vi "ADI_IMU_ADIS16448_GetSetRefNum.vi"(8 "error in (no error)":errorcluster, 9 "menu":enum16{"set", "get"}(ring), 10 "refnum name":string, 11 "ADI IMU Interrupt DevRef Set":T1) -> (0 "error out":errorcluster, 3 "ADI IMU Interrupt DevRef Get":T1)   [LabVIEW 2016, in "ADIS16448_IMU.lvlib"]
doc: "Sets a reference into a registry, gets a reference from a registry, or deletes a reference from a registry. The reference is accessed by name, and can be given any unique name.\n\nThis software is licensed. Open the labview\\readme\\WPI Robotics Library Open Source License.txt file for more information."
uses:
  ADIS16448_IMU.lvlib
  ADI_IMU_ADIS16448_InterruptDevRef.ctl
  ADI_IMU_ADIS16448_IMUDevRef.ctl
  <vilib>/Rock Robotics/SystemInterfaces/spilib/spi_bus.ctl
  <vilib>/Rock Robotics/WPI/Interrupt/WPI_InterruptRef.ctl
  <vilib>/Rock Robotics/SystemInterfaces/Interrupt/FPGA_InterruptIndex.ctl
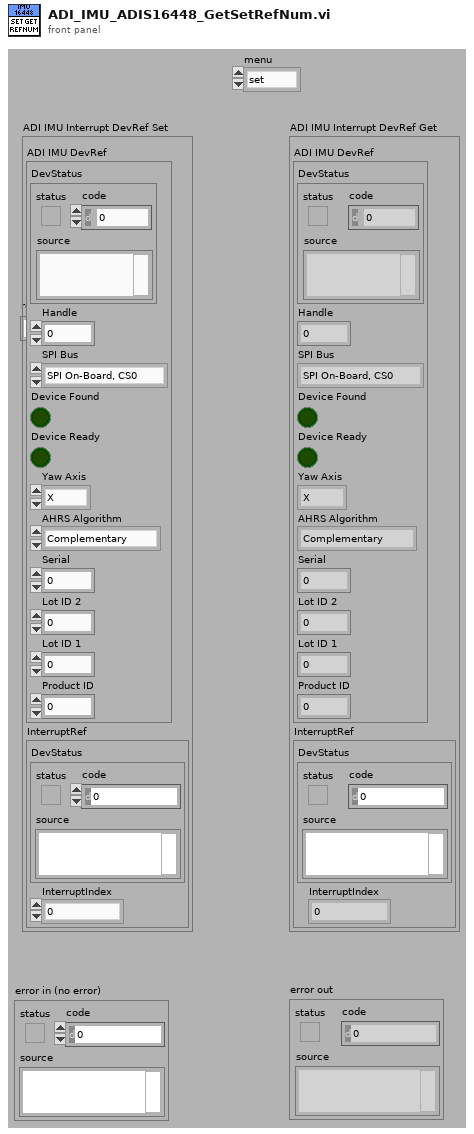
[diagram p1: front panel]
types:
  T1 = typedef "ADIS16448_IMU.lvlib/ADI_IMU_ADIS16448_InterruptDevRef.ctl" = cluster{"ADI IMU DevRef":T2, "InterruptRef":T4}
  T2 = typedef "ADIS16448_IMU.lvlib/ADI_IMU_ADIS16448_IMUDevRef.ctl" = cluster{"DevStatus":errorcluster, "Handle":i32, "SPI Bus":T3, "Device Found":bool, "Device Ready":bool, "Yaw Axis":enum16{"X", "Y", "Z"}, "AHRS Algorithm":enum16{"Complementary", "Madgwick"}, "Serial":u16, "Lot ID 2":u16, "Lot ID 1":u16, "Product ID":u16}
  T3 = typedef "spi_bus.ctl" = enum16{"SPI On-Board, CS0", "SPI On-Board, CS1", "SPI On-Board, CS2", "SPI On-Board, CS3", "SPI MXP", "Invalid"}
  T4 = typedef "WPI_InterruptRef.ctl" = cluster{"DevStatus":errorcluster, "InterruptIndex":T5}
  T5 = typedef "FPGA_InterruptIndex.ctl" = enum8{"0", "1", "2", "3", "4", "5", "6", "7", "Invalid"}
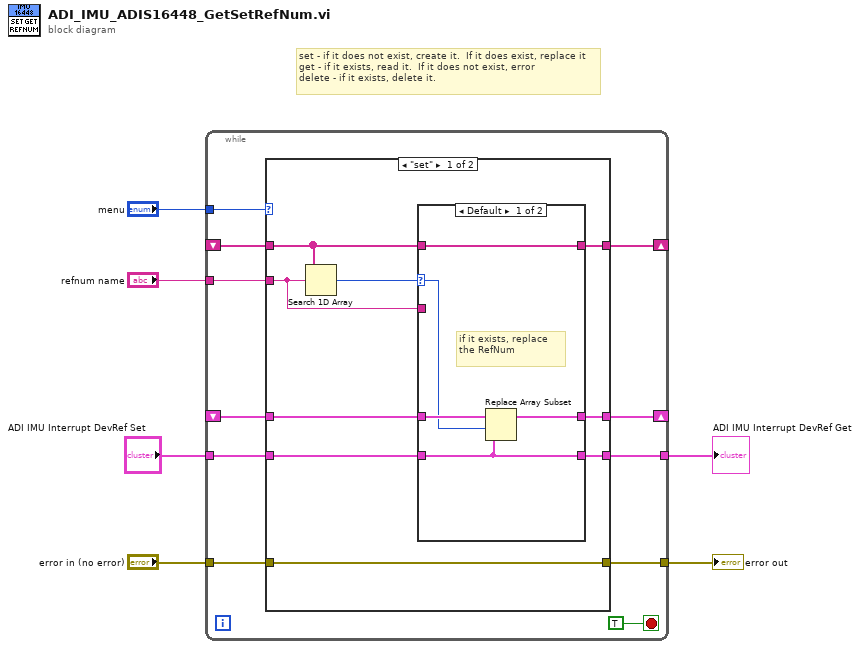
[diagram p0: block diagram]
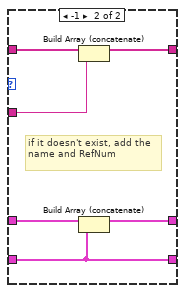
[diagram p2: hidden frame]
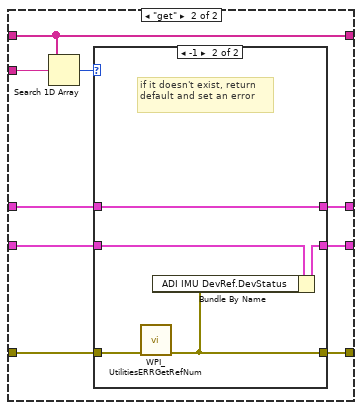
[diagram p3: hidden frame]
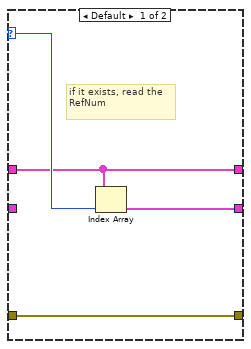
[diagram p4: hidden frame]
diagram:
  # "set - if it does not exist, create it.  If it does exist, replace it\nget - if it exists, read it.  If it does not exist, error\ndelete - if it exists, delete it."
  n1 = while {
    tunnel: "ADI IMU Interrupt DevRef Set" -> [w17]
    tunnel: "refnum name" -> [w10]
    tunnel: "error in (no error)" -> [w9]
    shift-right: [w16] -> _
    shift-left: _ -> [w15]
    tunnel: [w14] -> w1
    tunnel: "menu" -> [w13]
    shift-right: [w12] -> _
    shift-left: _ -> [w11]
    tunnel: [w8] -> w4
    stop <- TRUE stop-if-true
    n2 = case shown="\"set\"" w13 {
      tunnel: w17 -> [w21 w43]
      tunnel: [w20 w42] -> w16
      tunnel: w15 -> [w22 w44]
      tunnel: [w19 w41] -> w14
      tunnel: [w26 w40] -> w12
      tunnel: w11 -> [w25 w40]
      tunnel: w10 -> [w23 w45]
      tunnel: [w18 w38] -> w8
      tunnel: w9 -> [w18 w39]
      frame "set" {
        n3 = Search 1D Array(1D array=w25, element=w23) -> (index of element=w24:i32)  [unwired: 1 out]
        n4 = case shown="Default" w24 {
          selector: w24 -> [w29 _]
          tunnel: [w31 w37] -> w26
          tunnel: w25 -> [w31 w36]
          tunnel: w23 -> [_ w35]
          tunnel: w22 -> [w30 w34]
          tunnel: w21 -> [w27 w32]
          tunnel: [w28 w33] -> w20
          tunnel: [w27 w32] -> w19
          frame Default {
            # "if it exists, replace the RefNum"
            n5 = Replace Array Subset(array=w30, new element=w27, index=w29) -> (w28:T1[])
          }
          frame -1 {
            # "if it doesn't exist, add the name and RefNum"
            n6 = Build Array (concatenate)(w36, w35) -> (w37:string[])
            n7 = Build Array (concatenate)(w34, w32) -> (w33:T1[])
          }
        }
      }
      frame "get" {
        n8 = Search 1D Array(1D array=w40, element=w45) -> (index of element=w46:i32)  [unwired: 1 out]
        n9 = case shown="-1" w46 {
          selector: w46 -> [w50 _]
          tunnel: w44 -> [w48 w55]
          tunnel: w43 -> [_ w53]
          tunnel: [w48 w55] -> w42
          tunnel: [w49 w52] -> w41
          tunnel: w39 -> [w47 w54]
          tunnel: [w47 w51] -> w38
          frame Default {
            # "if it exists, read the RefNum"
            n10 = Index Array(array=w48, index=w50) -> (element=w49:T1)
          }
          frame -1 {
            # "if it doesn't exist, return default and set an error"
            n11 = call <vilib>:"WPI_UtilitiesERRGetRefNum.vi"("error in (no error)"=w54) -> ("ERRGetRefNum"=w51:errorcluster)  [unwired: 10 out]
            n12 = Bundle By Name(cluster=w53, "ADI IMU DevRef.DevStatus"=w51) -> (w52:T1)
          }
        }
      }
    }
  }
  "error out" <- w4
  "ADI IMU Interrupt DevRef Get" <- w1
